vi "Start Sync.vi"(8 "error in (no error)":errorcluster, 11 "gRPC Server in":refnum<class "TestService.lvclass">) -> (0 "error out":errorcluster, 3 "gRPC Server out":refnum<class "TestService.lvclass">)   [LabVIEW 2021, in "test_service_server.lvlib" / "TestService.lvclass"]
uses:
  TestService.lvclass
  TestService.lvclass/TestService.ctl
  test_service_server.lvlib
  RPC Messages/test_service_WaitResponse.ctl
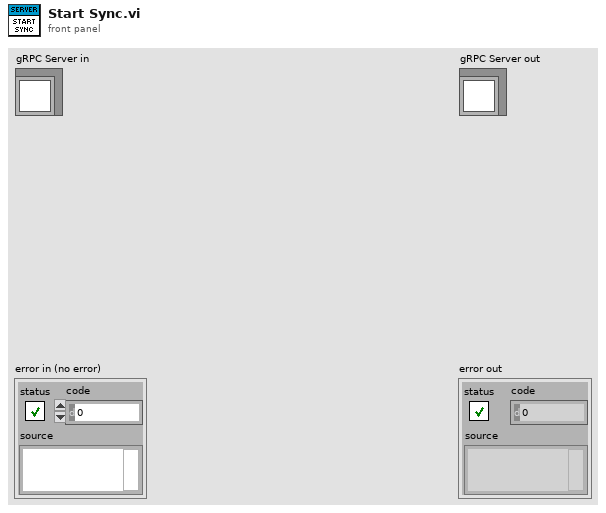
[diagram p1: front panel]
types:
  T1 = typedef "test_service_server.lvlib/test_service_WaitResponse.ctl" = cluster{"timestamp":u64}
  T2 = typedef "test_service_server.lvlib/TestService.lvclass/Server Internal UEs.ctl" = cluster{"TestService WaitMs Internal UE":refnum<user-event>}
  T3 = typedef "test_service_server.lvlib/TestService.lvclass/Server gRPC UEs.ctl" = cluster{"TestService WaitMs gRPC UE":refnum<user-event>}
  T4 = typedef "grpc-lvsupport-release.lvlib/grpcId.ctl" = u64
  T5 = typedef "test_service_server.lvlib/test_service_WaitRequest.ctl" = cluster{"msec_to_wait":u64}
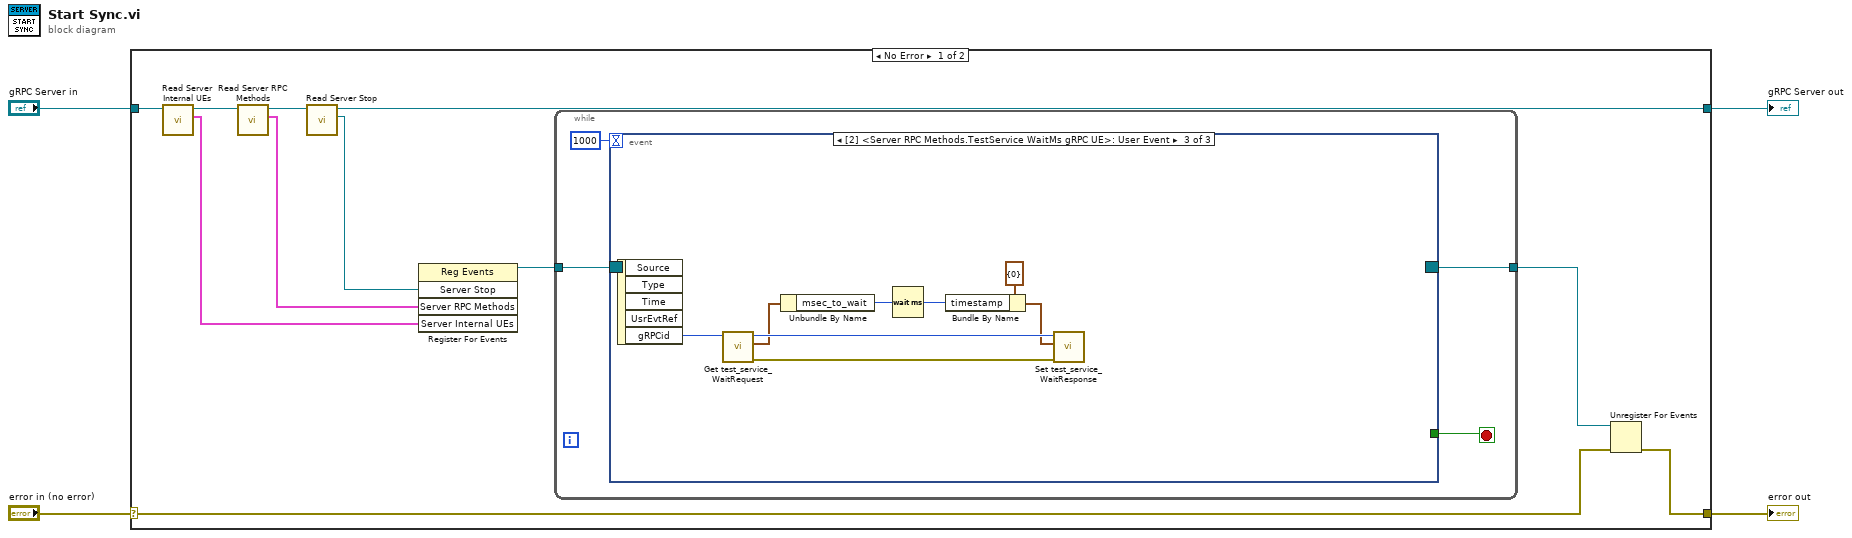
[diagram p0: block diagram]
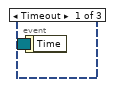
[diagram p2: hidden frame]
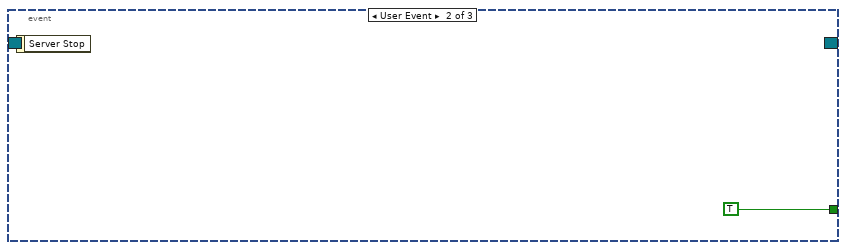
[diagram p3: hidden frame]
diagram:
  n1 = case shown="No Error" "error in (no error)" {
    selector: "error in (no error)" -> [w9 w30]
    tunnel: [w8 w30] -> w3
    tunnel: [w6 w29] -> w1
    tunnel: "gRPC Server in" -> [w15 w29]
    frame No Error {
      n2 = call "Read Server Internal UEs.vi"("SignalGeneratorService in"=w15) -> ("Server Internal UEs"=w13:T2, "SignalGeneratorService out"=w14:refnum<class "TestService.lvclass">)  [unwired: 8 in, 1 out]
      n3 = call "Read Server RPC Methods.vi"("SignalGeneratorService in"=w14) -> ("Server RPC Methods"=w7:T3, "SignalGeneratorService out"=w12:refnum<class "TestService.lvclass">)  [unwired: 8 in, 1 out]
      n4 = call-dynamic "Read Server Stop.vi"("iService in"=w12) -> ("Server Stop"=w5:refnum<user-event>, "iService out"=w6:refnum<class "TestService.lvclass">)  [unwired: 8 in, 1 out]
      n5 = register-events(w5, w7, w13) -> (reference out=w11:refnum<event-registration>)  [unwired: 2 in, 1 out]
      n6 = while {
        tunnel: w11 -> [w19]
        tunnel: [w17] -> w10
        stop <- w18 stop-if-true
        n7 = event "RPC Methods Event Structure" shown="[2] <Server RPC Methods.TestService WaitMs gRPC UE>: User Event" {
          selector: w19 -> [_ _ _]
          dyn-events: [_ _ _] -> w17
          timeout: 1000 -> [_ _ _]
          tunnel: [_ TRUE _] -> w18
          event Timeout {
            n8 = event-data() -> ()  [unwired: 1 in, 1 out]
          }
          event User Event {
            n9 = event-data() -> ()  [unwired: 1 in, 1 out]
          }
          event User Event {
            n10 = event-data() -> ("gRPCid"=w28:T4)  [unwired: 1 in, 4 out]
            n11 = call "Get test_service_WaitRequest.vi"("gRPCid"=w28) -> ("error out"=w21:errorcluster, "package_templatemessage"=w26:T5, "gRPCid out"=w27:T4)  [unwired: 8 in]
            n12 = Unbundle By Name(w26) -> ("msec_to_wait"=w24:u64)
            n13 = Wait (ms)(milliseconds to wait=w24) -> (millisecond timer value=w23:u32)
            n14 = Bundle By Name(cluster=T1 {"timestamp"=0} ("package_templatemessage"), "timestamp"=w23) -> (w22:T1)
            n15 = call "Set test_service_WaitResponse.vi"("error in (no error)"=w21, "package_templatemessage"=w22, "gRPCid"=w27) -> ()  [unwired: 8 in, 1 out]
          }
        }
      }
      n16 = Unregister For Events(event registration refnum=w10, error in=w9) -> (error out=w8:errorcluster)
    }
    frame Error {
    }
  }
  "error out" <- w3
  "gRPC Server out" <- w1
